vi "Advanced Remez Design with Exact Gain Control.vi"() -> ()   [LabVIEW 2023]
doc: "Demonstrates how to use the DFD Remez Design VI to design a finite impulse response (FIR) filter with frequency points of exact gain.\n\nComplete the following steps to use this VI.\n1) View the <B>Band Specifications</B> and <B>Sampling Frequency</B> controls to understand the pre-defined specifications of the filter design.\n2) Verify the <B>Apply Exact Gain Control?</B> value is off (FALSE).\n3) Run the VI. This VI designs an FIR filter with the pre-defined specifications and displays the magnitude response of the designed filter.\n4) Observe the <B>Basic Remez</B> plots on the Passband Magnitude Response and Stopband Magnitude Response. Notice that the magnitude response values are not 0 dB at DC and 500 Hz in the passband, and the magnitude response value is about -40 dB at 2.5 kHz in the stopband.\n5) Set the <B>Apply Exact Gain Control?</B> value to TRUE. This VI then uses the pre-defined specifications to design an FIR filter with frequency points of exact gain. The Frequency Points of Exact Gain section shows the controls that you can use to specify the frequency points of exact gain. Notice that this VI specifies two frequency points at DC and 500 Hz in the passband and one frequency point at 2.5 kHz in the stopband by default.\n6) Observe the <B>Advanced Remez</B> plots on the Passband Magnitude Response and Stopband Magnitude Response. Notice that the magnitude response values are 0 dB at DC and 500 Hz in the passband, and the magnitude response value is -Inf dB at 2.5 kHz in the stopband.\n7) Move the sliders in the Frequency Points of Exact Gain section to change the frequency points of exact gain and observe the <B>Advanced Remez</B> plots on the Passband Magnitude Response and Stopband Magnitude Response to find out the effects.\n8) Click the <B>STOP</B> button to stop this VI.\n9) Examine the block diagram to learn how to use the DFD Remez Design VI to design FIR filters with frequency points of exact gain."
uses:
  <vilib>/addons/Digital Filter Design/Analysis.llb/DFD Plot Freq Response (Linear-Spaced).vi
  <vilib>/addons/Digital Filter Design/NI_DigFilterLicensed.lvlib
panel:
  in  "Frequency Points of Exact Gain":T1={"Passband Frequency Point 1"=0.0, "Passband Frequency Point 2"=500.0, "Stopband Frequency Point"=2500.0} {"Stopband Frequency Point" scale=2000.0..5000.0 scale format="%_2p"; "Passband Frequency Point 2" scale=0.0..1000.0 scale format="%_2p"; "Passband Frequency Point 1" scale=0.0..1000.0 scale format="%_2p"}
  in  "Sampling Frequency":dbl=25000.0
  in  "Apply Exact Gain Control?":bool
  in  "stop":bool
  out "Stopband Magnitude Response":cluster{"f0":dbl, "df":dbl, "values":dbl[]}[](graph)
  out "Passband Magnitude Response":cluster{"f0":dbl, "df":dbl, "values":dbl[]}[](graph)
  in  "Orders":i32[](array[numeric])=[70, 78]
  in  "Band Specifications":T2(array[cluster])=[{"band specification"=[{"freq"=0.0, "amplitude"=1.0, "weight"=1.0}, {"freq"=1100.0, "amplitude"=1.0, "weight"=1.0}], "ripple constraint"=0.0}, {"band specification"=[{"freq"=1850.0, "amplitude"=0.0, "weight"=0.3}, {"freq"=12500.0, "amplitude"=0.0, "weight"=0.3}], "ripple constraint"=0.0}]
  # "Select Help>>Show Context Help and move the cursor over the VI icon for more information."
  # "frequency"
  # "amplitude"
  # "weight"
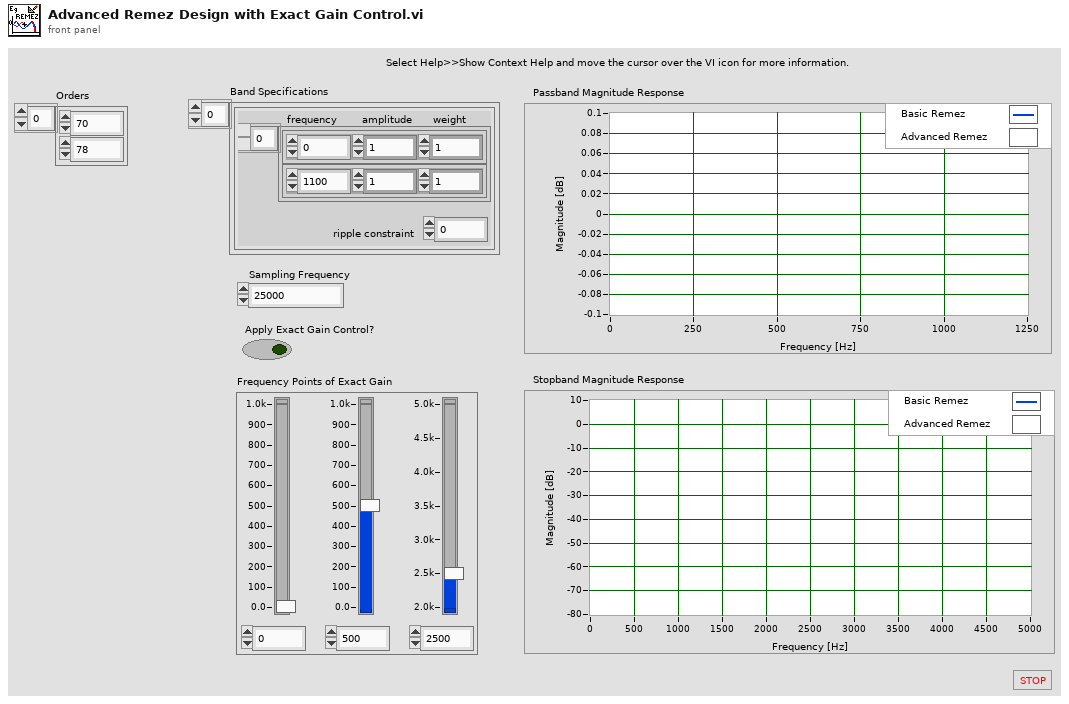
[diagram p1: front panel]
types:
  T1 = cluster{"Passband Frequency Point 1":dbl, "Passband Frequency Point 2":dbl, "Stopband Frequency Point":dbl}
  T2 = cluster{"band specification":cluster{"freq":dbl, "amplitude":dbl, "weight":dbl}[], "ripple constraint":dbl}[]
  T3 = typedef "NI_DigFilterLicensed.lvlib/DFD Filter Obj.ctl" = cluster{"mSRate_Fs":dbl, "mSRate_Version":string, "mSRate_Comments":string, "mSRate_OrgCoef":T4, "mSRate_CurCoef":T4, "mSRate_Quantized?":bool, "mSRate_QCoef":T4, "mSRate_QSettings":T6[], "mSRate_Order":i32, "mSRate_Scaling":cluster{"mSRate_ScaleByPowerOf2?":bool, "mSRate_ScaleType":T8}}
  T4 = typedef "NI_DigFilterLicensed.lvlib/DFD Filter Coef.ctl" = cluster{"type":T5, "gain":dbl, "coef a (k)":dbl[], "coef b (v)":dbl[]}
  T5 = typedef "NI_DigFilterLicensed.lvlib/DFD Filter Structure Type Selector.ctl" = enum16{"Undefined", "FIR Direct Form", "FIR Direct Form Transposed", "FIR Symmetric", "FIR Antisymmetric", "IIR Direct Form I", "IIR Direct Form I Transposed", "IIR Direct Form II", "IIR Direct Form II Transposed", "IIR Cascaded Second Order Sections Form I", "IIR Cascaded Second Order Sections Form I Transposed", "IIR Cascaded Second Order Sections Form II", "IIR Cascaded Second Order Sections Form II Transposed", "Lattice Allpass (basic sections)", "Lattice Allpass (one multiplier sections)", "Lattice Allpass (normalized sections)", "Lattice AR (basic sections)", "Lattice AR (one multiplier sections)", "Lattice AR (normalized sections)", "Lattice MA (minimum phase)", "Lattice MA (maximum phase)", "Lattice ARMA (basic sections)", "Lattice ARMA (one multiplier sections)", "Lattice ARMA (normalized sections)"}
  T6 = typedef "NI_DigFilterLicensed.lvlib/dfd_Internal Quantization Settings.ctl" = cluster{"source":T7, "wl":i16, "iwl":i16, "overflow mode":enum16{"Saturation", "Wrap"}, "rounding mode":enum16{"Nearest", "Truncation"}, "signed?":bool}
  T7 = typedef "NI_DigFilterLicensed.lvlib/dfd_Internal Quantization Srcs.ctl" = u16
  T8 = typedef "NI_DigFilterLicensed.lvlib/DFD Coef Norm Type.ctl" = enum16{"No Norm", "Time Domain 1-Norm", "Time Domain 2-Norm", "Time Domain Inf-Norm"}
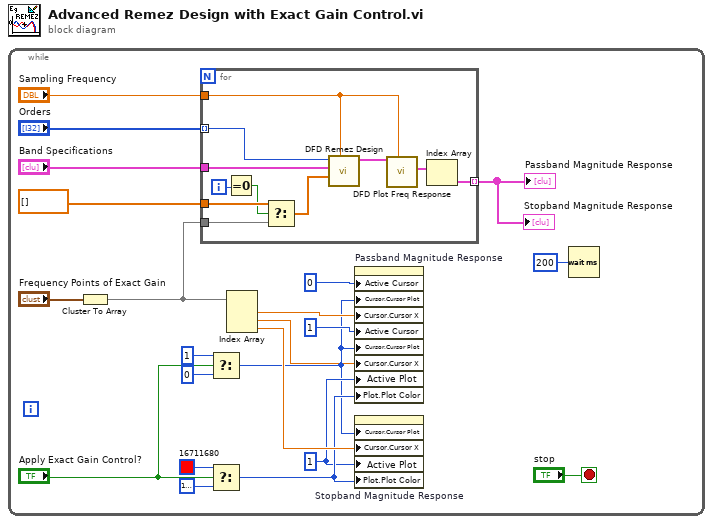
[diagram p0: block diagram]
diagram:
  n1 = while {
    stop <- "stop" stop-if-true
    w2 = u32 1 ("Active Plot")
    n2 = Cluster To Array(cluster="Frequency Points of Exact Gain") -> (array=w10:dbl[])
    n3 = for {
      tunnel: "Band Specifications" -> [w33]
      tunnel: "Orders" -> [w32] mode=indexing
      tunnel: dbl[] [] ("Array") -> [w31]
      tunnel: w10 -> [w30]
      tunnel: [w25] -> w19 mode=indexing
      tunnel: "Sampling Frequency" -> [w23]
      i -> [w29]
      n4 = Equal To 0?(x=w29) -> (x = 0?=w28:bool)
      n5 = Select(t=w31, s=w28, f=w30) -> (s? t:f=w27:dbl[])
      n6 = call <vilib>:"DFD Remez Design.vi"("fs [Hz]"=w23, "freqs of exact gain [Hz]"=w27, "band specs"=w33, "order"=w32) -> ("filter out"=w24:T3)  [unwired: 3 in, 4 out]
      n7 = call-poly <vilib>:"DFD Plot Freq Response.vi"("fs [Hz]"=w23, "filter in"=w24) -> ("magnitude response"=w26:cluster{"f0":dbl, "df":dbl, "values":dbl[]}[])  [unwired: 6 in, 3 out]
      n8 = Index Array(array=w26) -> (element=w25:cluster{"f0":dbl, "df":dbl, "values":dbl[]})  [unwired: 1 in]
    }
    "Passband Magnitude Response" <- w19
    "Stopband Magnitude Response" <- w19
    n9 = Select(t=1, s="Apply Exact Gain Control?", f=0 ("Cursor.Cursor Plot")) -> (s? t:f=w1:i32)
    n10 = Select(t=u32 16711680, s="Apply Exact Gain Control?", f=u32 16777216) -> (s? t:f=w8:u32)
    n11 = Index Array(array=w10) -> (element #1=w15:dbl, element #2=w14:dbl, element #3=w13:dbl)  [unwired: 3 in]
    n12 = property on="Passband Magnitude Response" class="WFGraph (strict)"("Active Cursor"=u32 0, "Cursor.Cursor Plot"=w1, "Cursor.Cursor X"=w15, "Active Cursor"=u32 1, "Cursor.Cursor Plot"=w1, "Cursor.Cursor X"=w14, "Active Plot"=w2, "Plot.Plot Color"=w8) -> ()  [unwired: 2 in, 2 out]
    n13 = property on="Stopband Magnitude Response" class="WFGraph (strict)"("Cursor.Cursor Plot"=w1, "Cursor.Cursor X"=w13, "Active Plot"=w2, "Plot.Plot Color"=w8) -> ()  [unwired: 2 in, 2 out]
    n14 = Wait (ms)(milliseconds to wait=u32 200) -> ()  [unwired: 1 out]
  }
